vi "RootGraph.vi"() -> ()   [LabVIEW 2013, in "PanelRootNode.lvclass"]
uses:
  PanelRootNode.lvclass
  PanelObject/PanelObject.lvclass
  PanelDataNode/PanelDataNode.lvclass
  PanelDataNode/PanelDataNode.lvclass/PanelDataNode.ctl
  PanelDataNode/Split Mode.ctl
  <vilib>/Analysis/baseanly.llb/Mean (DBL).vi
  PanelLinkNode/PanelLinkNode.lvclass
  share/QueueManager.llb/Insert.vi
  <vilib>/measure/NI_MABase.lvlib
  <vilib>/Analysis/NI_AALBase.lvlib
panel:
  in  "signal type":T1(ring) caption="信号类型"
  in  "Node*":refnum<data-value>
  out "波形图表":waveform(dbl)(graph)={"t0"=timestamp(9406.0 s since 1904-01-01), "dt"=0.001, "Y"=array[1000 elements]}
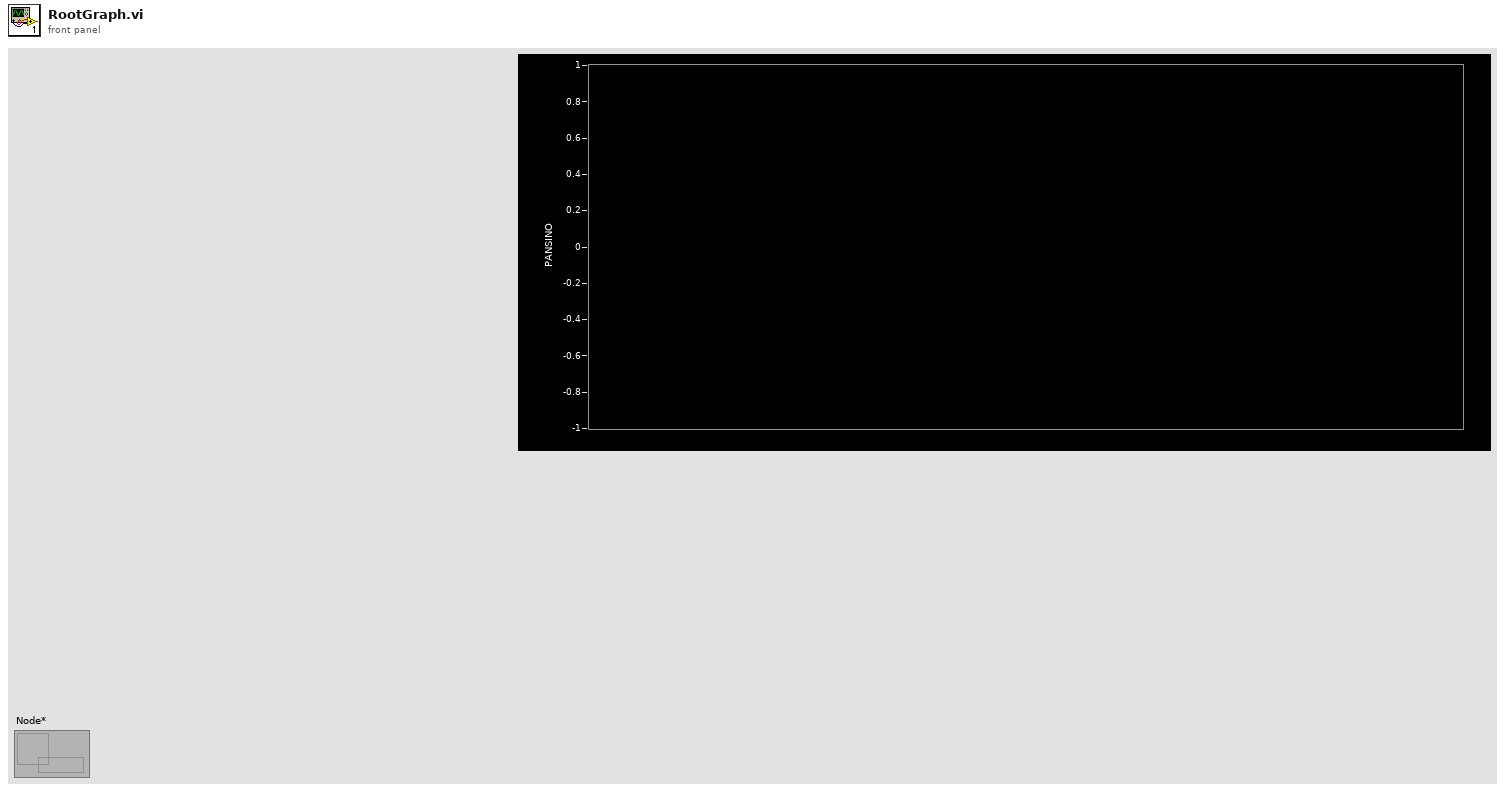
[diagram p1: front panel]
types:
  T1 = enum16{"Sine Wave", "Triangle Wave", "Square Wave", "Sawtooth Wave"}
  T2 = typedef "PanelDataNode.lvclass/Split Mode.ctl" = enum16{"Horizontal(up)", "Vertical(left)", "Horizontal(down)", "Vertical(right)"}
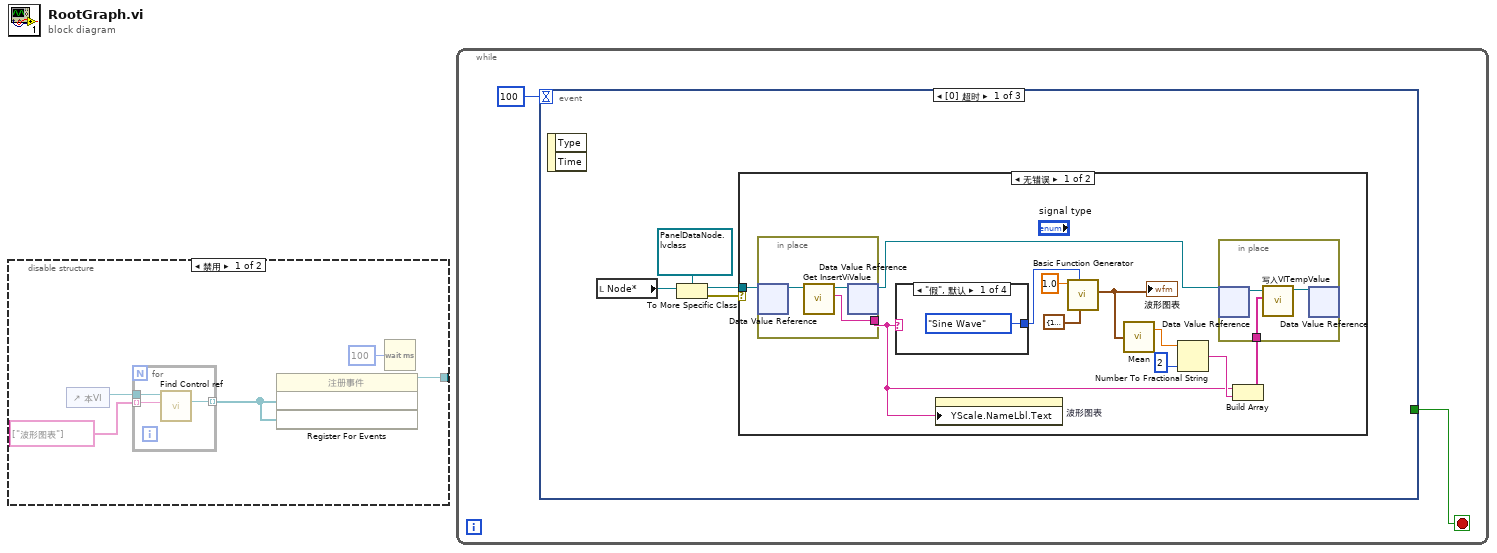
[diagram p0: block diagram]
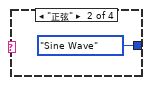
[diagram p3: hidden frame]
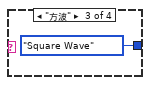
[diagram p4: hidden frame]
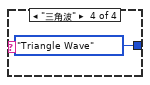
[diagram p5: hidden frame]
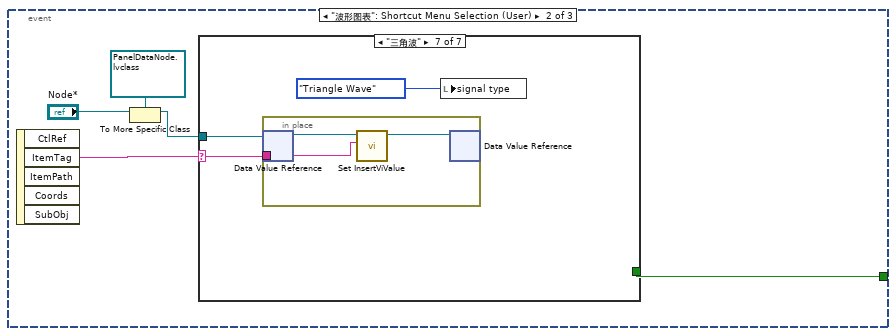
[diagram p7: hidden frame]
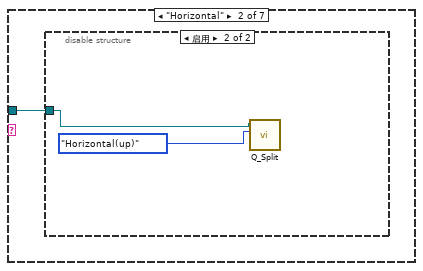
[diagram p9: hidden frame]
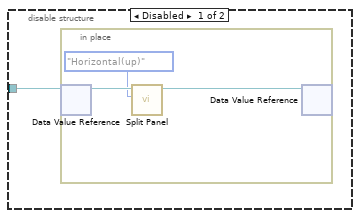
[diagram p10: hidden frame]
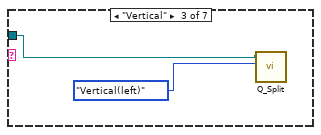
[diagram p11: hidden frame]
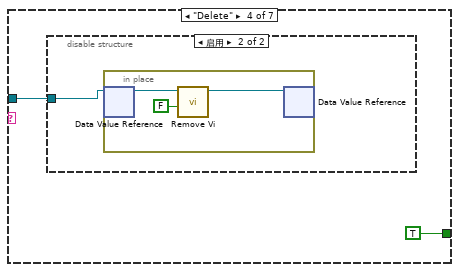
[diagram p12: hidden frame]
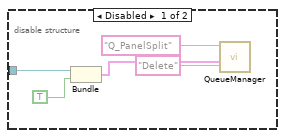
[diagram p13: hidden frame]
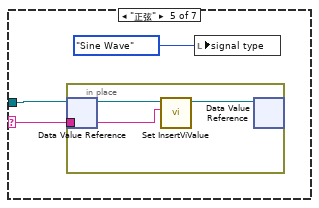
[diagram p14: hidden frame]
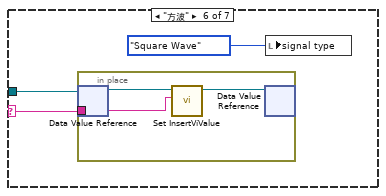
[diagram p15: hidden frame]
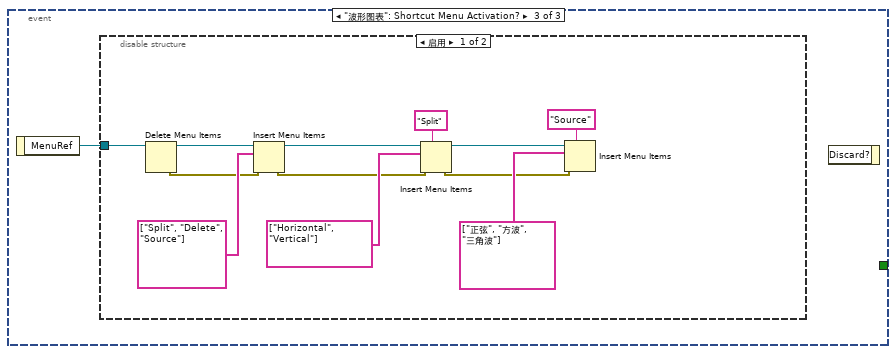
[diagram p16: hidden frame]
diagram:
  n1 = disable-structure shown="禁用" {
    disable-tunnel: [w3 _] -> _
    frame Disabled {
      n2 = control-ref of="本VI"() -> (w5:refnum<vi>)
      n3 = for {
        tunnel: w5 -> [w8]
        tunnel: string[] ["波形图表"] -> [w7] mode=indexing
        tunnel: [w6] -> w2 mode=indexing
        n4 = call "Find Control ref.vi"("control name"=w7, "panelvi*"=w8) -> ("ctrl*"=w6:refnum<vi>)  [unwired: 7 in, 2 out]
      }
      n5 = register-events(w2, w2) -> (reference out=w3:refnum<event-registration>)  [unwired: 2 in, 1 out]
      n6 = Wait (ms)(milliseconds to wait=u32 100 ("等待时间（毫秒）")) -> ()  [unwired: 1 out]
    }
    frame Enabled {
    }
  }
  n7 = while {
    stop <- w9 stop-if-true
    n8 = event shown="[0] 超时" {
      selector: _ -> [_ _ _]
      dyn-events: _ -> [_ _ _]
      timeout: 100 -> [_ _ _]
      tunnel: [_ w36 _] -> w9
      event Timeout {
        n9 = event-data() -> ()  [unwired: 1 in, 2 out]
        n10 = local read "Node*"() -> (w13:refnum<data-value>)
        n11 = To More Specific Class(target class=refnum<data-value> refnum ("Node*"), reference=w13) -> (specific class reference=w11:refnum<data-value>, error out=w12:errorcluster)  [unwired: 1 in]
        n12 = case shown="无错误" w12 {
          tunnel: w11 -> [w23 _]
          frame No Error {
            n13 = in-place {
              in-place-border: [w33] -> w15
              n14 = in-place-dvr #1(w23) -> (w35:refnum<class "PanelDataNode.lvclass">)  [unwired: 1 out]
              n15 = call-dynamic "Get InsertViValue.vi"("PanelDataNode 输入"=w35) -> ("ViValue"=w33:string, "PanelDataNode 输出"=w34:refnum<class "PanelDataNode.lvclass">)  [unwired: 8 in, 1 out]
              n16 = in-place-dvr #1(w34) -> (w20:refnum<data-value>)  [unwired: 1 out]
            }
            n17 = case shown="\"假\", 默认" w15 {
              tunnel: [T1."Sine Wave" ("signal type") T1."Sine Wave" ("signal type") T1."Square Wave" ("signal type") T1."Triangle Wave" ("signal type")] -> w22
              frame "假", Default {
              }
              frame "正弦" {
              }
              frame "方波" {
              }
              frame "三角波" {
              }
            }
            n18 = property on="波形图表" class="WFChart (严格)"("YScale.NameLbl.Text"=w15) -> ()  [unwired: 2 in, 2 out]
            n19 = call <vilib>:"Basic Function Generator.vi"("sampling info"=cluster{"Fs":dbl, "#s":dbl} {"Fs"=100.0, "#s"=101.0}, "signal type"=w22, "frequency"=1.0) -> ("signal out"=w21:waveform(dbl))  [unwired: 6 in, 2 out]
            "波形图表" <- w21
            n20 = call-poly <vilib>:"Mean.vi"("X"=w21) -> ("mean"=w19:dbl)  [unwired: 1 out]
            n21 = Number To Fractional String(number=w19, precision (6)=i16 2 ("精度(6)")) -> (F-format string=w17:string)  [unwired: 2 in]
            n22 = Build Array(w15, w17) -> (w16:string[])
            n23 = in-place {
              in-place-border: w16 -> [w26]
              n24 = in-place-dvr #2(w20) -> (w28:refnum<class "PanelDataNode.lvclass">)  [unwired: 1 out]
              n25 = call "写入VITempValue.vi"("VITempValue"=w26, "PanelDataNode输入"=w28) -> ("PanelDataNode输出"=w27:refnum<class "PanelDataNode.lvclass">)  [unwired: 8 in, 1 out]
              n26 = in-place-dvr #2(w27) -> ()  [unwired: 2 out]
            }
          }
          frame Error {
          }
        }
      }
      event "波形图表": Shortcut Menu Selection (User) {
        n27 = event-data() -> ("ItemTag"=w40:string)  [unwired: 1 in, 4 out]
        n28 = To More Specific Class(target class=refnum<data-value> refnum ("Node*"), reference="Node*") -> (specific class reference=w37:refnum<data-value>)  [unwired: 1 in, 1 out]
        n29 = case shown="\"三角波\"" w40 {
          selector: w40 -> [_ _ _ _ w61 w67 w73]
          tunnel: w37 -> [_ w41 w49 w50 w62 w68 w74]
          tunnel: [_ _ _ TRUE _ _ _] -> w36
          frame "假", Default {
          }
          frame "Horizontal" {
            n30 = disable-structure shown="启用" {
              disable-tunnel: w41 -> [w42 w47]
              frame Disabled {
                n31 = in-place {
                  n32 = in-place-dvr #3(w42) -> (w45:refnum<class "PanelDataNode.lvclass">)  [unwired: 1 out]
                  n33 = call-dynamic "Split Panel.vi"("Split Mode"=Split_Mode."Horizontal(up)", "PanelDataNode 输入"=w45) -> ("PanelDataNode 输出"=w44:refnum<class "PanelDataNode.lvclass">)  [unwired: 7 in, 2 out]
                  n34 = in-place-dvr #3(w44) -> ()  [unwired: 2 out]
                }
              }
              frame Enabled {
                n35 = call "Q_Split.vi"("Split Mode"=Split_Mode."Horizontal(up)", "ChildNode*"=w47) -> ()  [unwired: 9 in, 1 out]
              }
            }
          }
          frame "Vertical" {
            n36 = call "Q_Split.vi"("Split Mode"=Split_Mode."Vertical(left)", "ChildNode*"=w49) -> ()  [unwired: 9 in, 1 out]
          }
          frame "Delete" {
            n37 = disable-structure shown="启用" {
              disable-tunnel: w50 -> [w56 w57]
              frame Disabled {
                n38 = Bundle("Node*"=w56, TRUE) -> (w54:cluster{"Node*":refnum<data-value>, bool})  [unwired: 1 in]
                n39 = call-poly "QueueManager.vi"("Data"=w54, "Event"="Delete", "QueueName"="Q_PanelSplit") -> ()  [unwired: 7 in, 2 out]
              }
              frame Enabled {
                n40 = in-place {
                  n41 = in-place-dvr #4(w57) -> (w60:refnum<class "PanelDataNode.lvclass">)  [unwired: 1 out]
                  n42 = call-dynamic "Remove Vi.vi"("Abort VI"=FALSE, "PanelDataNode 输入"=w60) -> ("PanelDataNode 输出"=w59:refnum<class "PanelDataNode.lvclass">)  [unwired: 6 in, 3 out]
                  n43 = in-place-dvr #4(w59) -> ()  [unwired: 2 out]
                }
              }
            }
          }
          frame "正弦" {
            n44 = in-place {
              in-place-border: w61 -> [w65]
              n45 = in-place-dvr #5(w62) -> (w66:refnum<class "PanelDataNode.lvclass">)  [unwired: 1 out]
              n46 = call-dynamic "Set InsertViValue.vi"("ViValue"=w65, "PanelDataNode 输入"=w66) -> ("PanelDataNode 输出"=w64:refnum<class "PanelDataNode.lvclass">)  [unwired: 8 in, 1 out]
              n47 = in-place-dvr #5(w64) -> ()  [unwired: 2 out]
            }
            n48 = local write "signal type"(T1."Sine Wave" ("signal type")) -> ()
          }
          frame "方波" {
            n49 = in-place {
              in-place-border: w67 -> [w71]
              n50 = in-place-dvr #6(w68) -> (w72:refnum<class "PanelDataNode.lvclass">)  [unwired: 1 out]
              n51 = call-dynamic "Set InsertViValue.vi"("ViValue"=w71, "PanelDataNode 输入"=w72) -> ("PanelDataNode 输出"=w70:refnum<class "PanelDataNode.lvclass">)  [unwired: 8 in, 1 out]
              n52 = in-place-dvr #6(w70) -> ()  [unwired: 2 out]
            }
            n53 = local write "signal type"(T1."Square Wave" ("signal type")) -> ()
          }
          frame "三角波" {
            n54 = in-place {
              in-place-border: w73 -> [w77]
              n55 = in-place-dvr #7(w74) -> (w78:refnum<class "PanelDataNode.lvclass">)  [unwired: 1 out]
              n56 = call-dynamic "Set InsertViValue.vi"("ViValue"=w77, "PanelDataNode 输入"=w78) -> ("PanelDataNode 输出"=w76:refnum<class "PanelDataNode.lvclass">)  [unwired: 8 in, 1 out]
              n57 = in-place-dvr #7(w76) -> ()  [unwired: 2 out]
            }
            n58 = local write "signal type"(T1."Triangle Wave" ("signal type")) -> ()
          }
        }
      }
      event "波形图表": Shortcut Menu Activation? {
        n59 = event-data() -> ("MenuRef"=w79:refnum<k9>)  [unwired: 1 in]
        n60 = disable-structure shown="启用" {
          disable-tunnel: w79 -> [w91 _]
          frame Enabled {
            n61 = Delete Menu Items(9:w91) -> (0:w82:errorcluster, 3:w90:refnum<k9>)  [unwired: 3 in]
            n62 = Insert Menu Items(6:w82, 8:string[] ["Split", "Delete", "Source"] ("项名称"), 9:w90) -> (0:w81:errorcluster, 3:w88:refnum<k9>)  [unwired: 3 in, 1 out]
            n63 = Insert Menu Items(5:"Split" ("菜单标识符"), 6:w81, 8:string[] ["Horizontal", "Vertical"], 9:w88) -> (0:w80:errorcluster, 3:w85:refnum<k9>)  [unwired: 2 in, 1 out]
            n64 = Insert Menu Items(5:"Source" ("菜单标识符"), 6:w80, 8:string[] ["正弦", "方波", "三角波"] ("项名称"), 9:w85) -> ()  [unwired: 2 in, 3 out]
          }
          frame Disabled {
          }
        }
        n65 = event-data() -> ()  [unwired: 2 in, 1 out]
      }
    }
  }
